vi "Set Impulse Positions.vi"(10 "Impulse Positions":T2(array[cluster]) {"Amplitude offset" format="%.2f"}, 11 "Reference in":T1) -> (3 "Reference out":T1)   [LabVIEW 2016, in "Impulse Data.lvclass"]
uses:
  Impulse Data.lvclass
  Instance handle.ctl
  Impulse Data.lvclass/Impulse Data.ctl
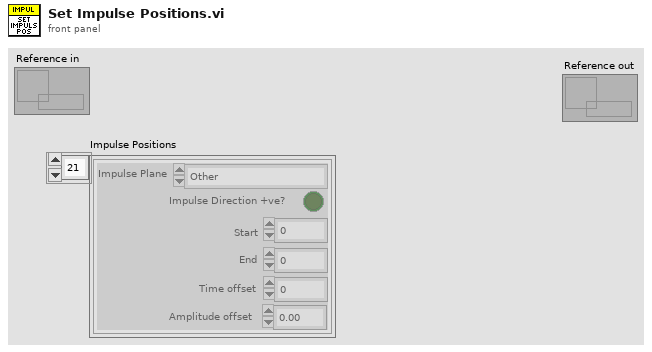
[diagram p1: front panel]
types:
  T1 = typedef "Impulse Data.lvclass/Instance handle.ctl" = refnum<data-value>
  T2 = cluster{"Start":i32, "End":i32, "Impulse Plane":enum16{"Other", "Yaw", "Pitch", "Roll", "LARP", "RALP"}, "Impulse Direction +ve?":bool, "Time offset":i32, "Amplitude offset":dbl}[]
  T3 = typedef "TD_Impulse Planes.ctl" = enum16{"Other", "Yaw", "Pitch", "Roll", "LARP", "RALP"}
  T4 = cluster{"Impulse Plane":T3, "Impulse Direction +ve?":bool, "Start":i32, "Duration":i32}[]
  T5 = cluster{"Impulse Plane":T3, "Impulse Direction +ve?":bool, "Start":i32, "Duration":i32}
  T6 = enum16{"Other", "Yaw", "Pitch", "Roll", "LARP", "RALP"}
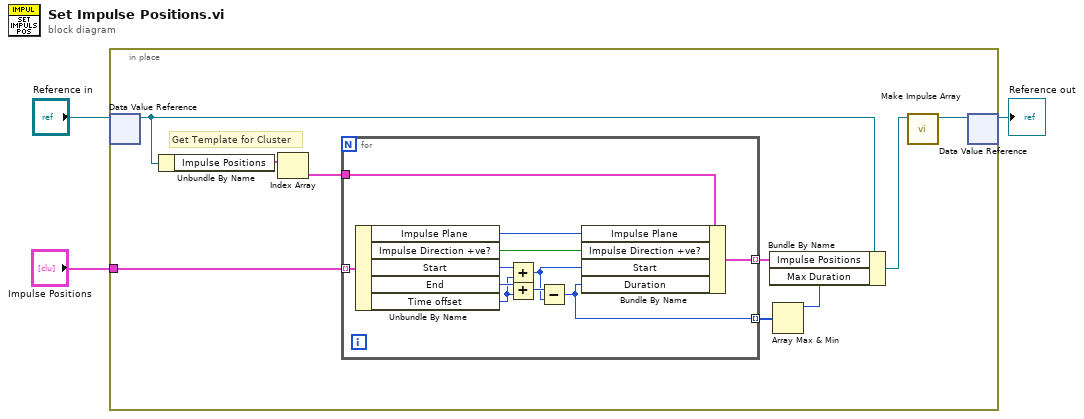
[diagram p0: block diagram]
diagram:
  n1 = in-place {
    in-place-border: "Impulse Positions" -> [w12]
    # "Get Template for Cluster"
    n2 = in-place-dvr #1("Reference in") -> (w4:refnum<class "Impulse Data.lvclass">)  [unwired: 1 out]
    n3 = Unbundle By Name(w4) -> ("Impulse Positions"=w11:T4)
    n4 = Index Array(array=w11) -> (element=w10:T5)  [unwired: 1 in]
    n5 = for {
      tunnel: w12 -> [w23] mode=indexing
      tunnel: w10 -> [w18]
      tunnel: [w14] -> w9 mode=indexing
      tunnel: [w13] -> w8 mode=indexing
      n6 = Unbundle By Name(w23) -> ("Impulse Plane"=w17:T6, "Impulse Direction +ve?"=w16:bool, "Start"=w21:i32, "End"=w20:i32, "Time offset"=w19:i32)
      n7 = Add(x=w21, y=w19) -> (x+y=w15:i32)
      n8 = Add(x=w20, y=w19) -> (x+y=w22:i32)
      n9 = Subtract(x=w22, y=w15) -> (x-y=w13:i32)
      n10 = Bundle By Name(cluster=w18, "Impulse Plane"=w17, "Impulse Direction +ve?"=w16, "Start"=w15, "Duration"=w13) -> (w14:T5)
    }
    n11 = Array Max & Min(array=w8) -> (max value=w7:i32)  [unwired: 3 out]
    n12 = Bundle By Name(cluster=w4, "Impulse Positions"=w9, "Max Duration"=w7) -> (w6:refnum<class "Impulse Data.lvclass">)
    n13 = call "Make Impulse Array.vi"("Class out"=w6) -> ("Class In"=w5:refnum<class "Impulse Data.lvclass">)  [unwired: 9 in, 1 out]
    n14 = in-place-dvr #1(w5) -> (→"Reference out":T1)  [unwired: 1 out]
  }
